vi "db_connectv2.vi"() -> ()   [LabVIEW 2016]
uses:
  <vilib>/addons/database/Connection.llb/DB Tools Open Connec (Path).vi
  <vilib>/addons/database/NI_Database_API.lvlib
panel:
  in  "OK Button":bool
  in  "data insert":T1={"Descrição"="Descrição", "Tensão"=0, "Capacidade"=0}
  out "data ensaio":string[][](table)
  in  "Table ID":u16(ring) items=["Bateria Unipower 1", "Bateria Unipower 2", "Bateria Unipower 3", "Bateria Unipower 4", "Bateria Unipower 5", "Bateria Unipower 6", "Bateria Unipower 7", "Bateria Unipower 8", "Bateria Unipower 9", "Bateria Unipower 10"]
  out "data bateria":string[][](table)
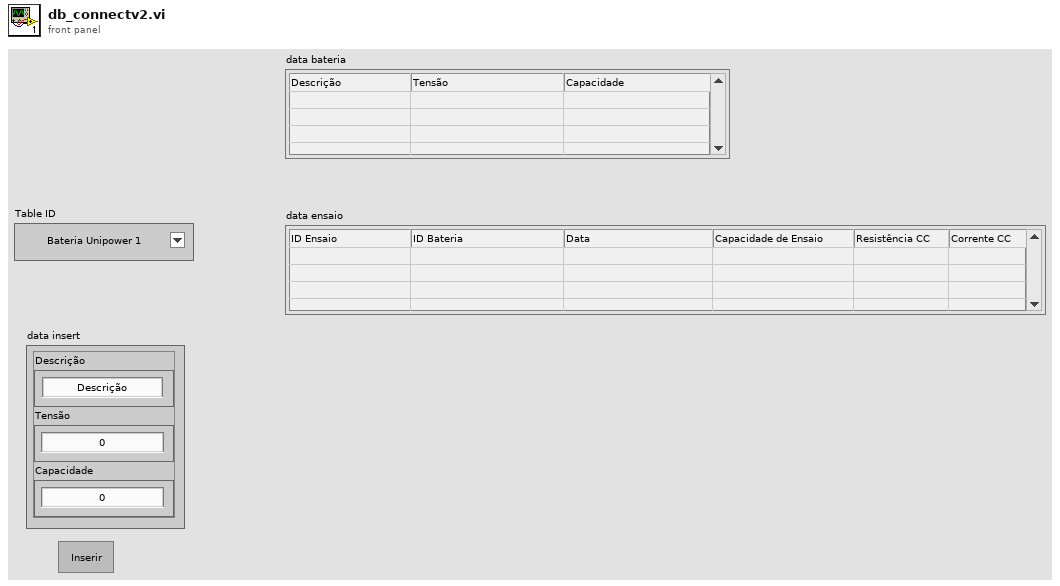
[diagram p1: front panel]
types:
  T1 = cluster{"Descrição":string, "Tensão":i32, "Capacidade":i32}
  T2 = typedef "NI_Database_API.lvlib/Conn ObjectReference.ctl" = refnum<k1>
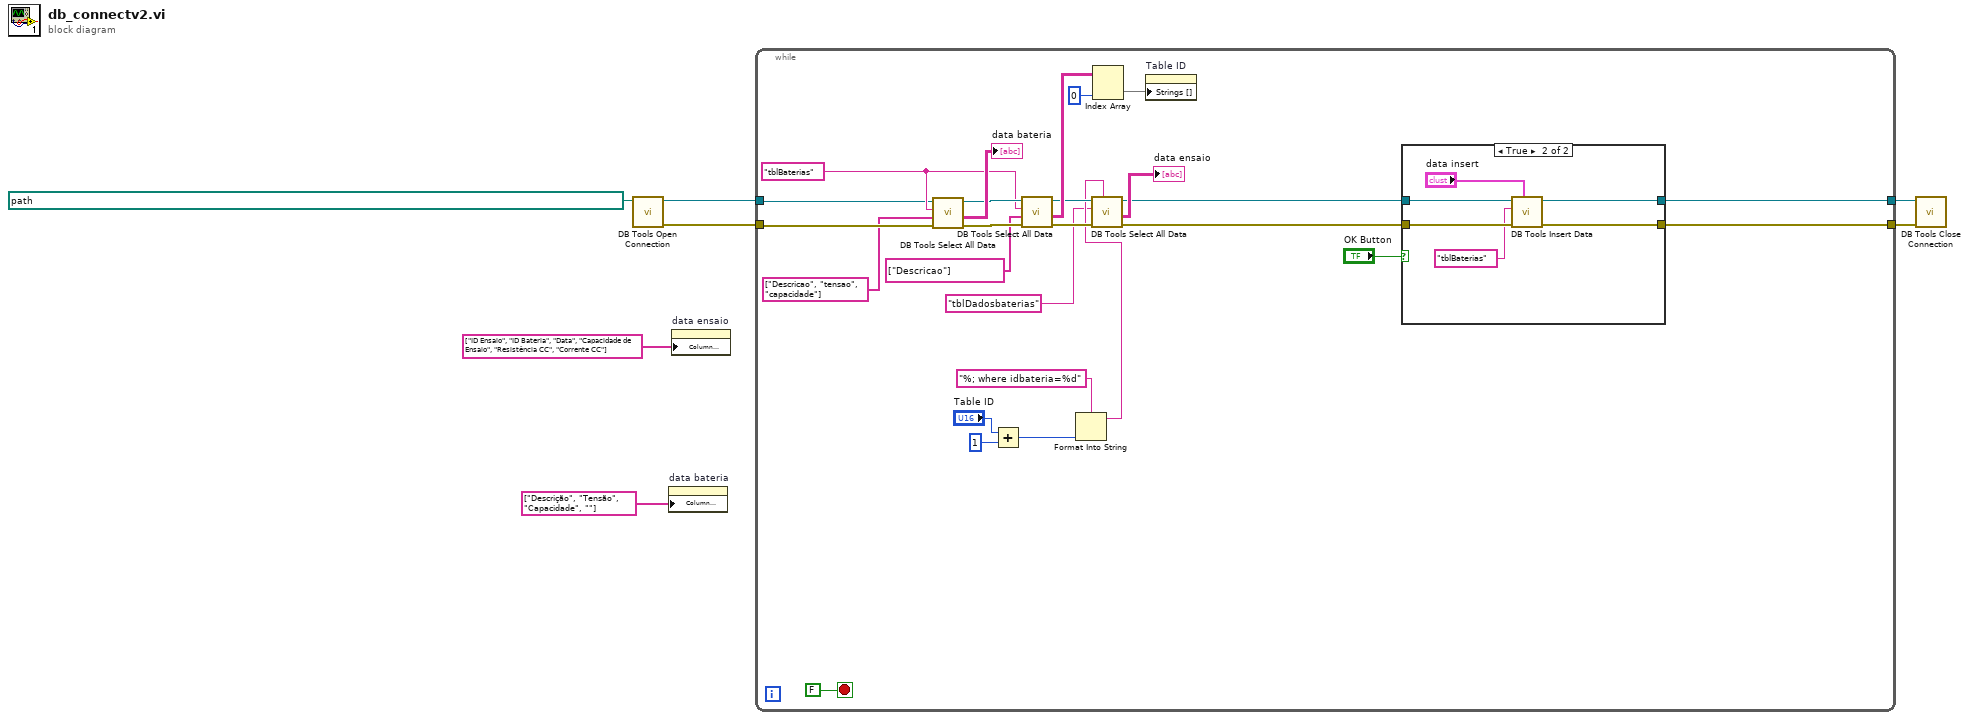
[diagram p0: block diagram]
diagram:
  n1 = call-poly <vilib>:"DB Tools Open Connection.vi"("connection information"=path "D:/UFSM/Engenharia de Controle e Automação/8 Semestre/Projeto Integrador - DPEE 1064/LabVIEW/database.udl") -> ("error out"=w3:errorcluster, "connection reference"=w4:T2)  [unwired: 7 in]
  n2 = property on="data bateria" class="Tbl (strict)"("Column Headers[]"=string[] ["Descrição", "Tensão", "Capacidade", ""] ("Column Header Strings[]")) -> ()  [unwired: 2 in, 2 out]
  n3 = property on="data ensaio" class="Tbl (strict)"("Column Headers[]"=string[] ["ID Ensaio", "ID Bateria", "Data", "Capacidade de Ensaio", "Resistência CC", "Corrente CC"] ("columns")) -> ()  [unwired: 2 in, 2 out]
  n4 = while {
    tunnel: w3 -> [w16]
    tunnel: w4 -> [w17]
    tunnel: [w11] -> w7
    tunnel: [w9] -> w6
    stop <- FALSE stop-if-true
    w29 = "tblBaterias" ("table")
    n5 = call <vilib>:"DB Tools Select All Data.vi"("error in (no error)"=w16, "columns"=string[] ["Descricao", "tensao", "capacidade"], "table"=w29, "connection reference"=w17) -> ("error out"=w31:errorcluster, "data"=→"data bateria":string[][], "connection reference out"=w30:T2)  [unwired: 2 in]
    n6 = Add(x="Table ID", y=u16 1) -> (x+y=w19:u16)
    n7 = call <vilib>:"DB Tools Select All Data.vi"("error in (no error)"=w31, "columns"=string[] ["Descricao"], "table"=w29, "connection reference"=w30) -> ("error out"=w23:errorcluster, "data"=w26:string[][], "connection reference out"=w24:T2)  [unwired: 2 in]
    n8 = Format Into String(format string="%; where idbateria=%d" ("condition"), w19) -> (resulting string=w21:string)  [unwired: 2 in, 1 out]
    n9 = call <vilib>:"DB Tools Select All Data.vi"("optional clause"=w21, "error in (no error)"=w23, "table"="tblDadosbaterias", "connection reference"=w24) -> ("error out"=w10:errorcluster, "data"=→"data ensaio":string[][], "connection reference out"=w12:T2)  [unwired: 2 in]
    n10 = Index Array(array=w26, index (col)=0 ("disabled index (col)")) -> (element=w25:string[])  [unwired: 1 in]
    n11 = property on="Table ID" class="Ring (strict)"("Strings []"=w25) -> ()  [unwired: 2 in, 2 out]
    n12 = case shown="True" "OK Button" {
      tunnel: w12 -> [w35 w41]
      tunnel: [w35 w40] -> w11
      tunnel: w10 -> [w34 w39]
      tunnel: [w34 w38] -> w9
      frame False {
      }
      frame True {
        n13 = call <vilib>:"DB Tools Insert Data.vi"("data"="data insert", "error in (no error)"=w39, "table"="tblBaterias", "connection reference"=w41) -> ("error out"=w38:errorcluster, "connection reference out"=w40:T2)  [unwired: 6 in]
      }
    }
  }
  n14 = call <vilib>:"DB Tools Close Connection.vi"("error in (no error)"=w6, "connection reference"=w7) -> ()  [unwired: 5 in, 1 out]
